vi "String to Cluster.vi"(1 "string":string) -> (0 "Correlator Initial Data 2":T1={"[0]"=1, "Channel1 Threshold Voltage (mV)"=1, "Channel1 Pulse Front"="", "Channel2 Threshold Voltage (mV)"=1, "Channel2 Pulse Front"="", "Channel3 Threshold Voltage (mV)"=1, "Channel3 Pulse Front "="", "Channel4 Threshold Voltage (mV)"=1, "Channel4 Pulse Front "="", "Single Count Enable"={"Channel1"=FALSE, "Channel2"=FALSE, "Channel3"=FALSE, "Channel4"=FALSE}, "Single Count Max"=1, "Sum Count Enable"={"Channel1"=FALSE, "Channel2"=FALSE, "Channel3"=FALSE, "Channel4"=FALSE}, "Sum Count Max"=1, "Start-Stop1 Multyplex"={"Stop Channel"="", "Start Channel"=""}, "Stop Delay 1 (ns)"=1, "Window Length 1 (ns)"=4, "Window Offset 1 (ns) "=4, "Conditional Correlation 1"="", "Histogram Bin 1"="", "Histogram Start 1 (ns) "=4, "Start-Stop2 Multyplex "={"Stop Channel"="", "Start Channel"=""}, "Stop Delay 2 (ns)"=1, "Window Length 2 (ns) "=4, "Window Offset 2 (ns) "=4, "Conditional Correlation 2"="", "Histogram Bin 2"="", "Histogram Start 2 (ns)  "=4, "Start-Stop3 Multyplex"={"Stop Channel"="", "Start Channel"=""}, "Stop Delay 3 (ns)"=1, "Window Length 3 (ns) "=4, "Window Offset 3 (ns) "=4, "Conditional Correlation 3"="", "Histogram Bin 3"="", "Histogram Start 3 (ns) "=4, "Start-Stop4 Multyplex"={"Stop Channel"="", "Start Channel"=""}, "Stop Delay 4 (ns)"=1, "Window Length 4 (ns)  "=4, "Window Offset 4 (ns) "=4, "Conditional Correlation 4"="", "Histogram Bin 4"="", "Histogram Start 4 (ns)  "=4, "Coincidence Count Enable"={"Start-Stop1"=FALSE, "Start-Stop2"=FALSE, "Start-Stop3"=FALSE, "Start-Stop4"=FALSE}, "Coincidence Count Max"=1, "Coincidence Sum Enable"={"Start-Stop1"=FALSE, "Start-Stop2"=FALSE, "Start-Stop3"=FALSE, "Start-Stop4"=FALSE}, "Coincidence Sum Max"=1, "Output Channel Enable"={"Channel1"=FALSE, "Channel2"=FALSE, "Channel3"=FALSE, "Channel4"=FALSE}, "Output Channel Inversion"={"Channel1"=FALSE, "Channel2"=FALSE, "Channel3"=FALSE, "Channel4"=FALSE, "Output"=FALSE}} {"Coincidence Sum Max" min=1 max=16777215 step=1 format="%.7e"; "Coincidence Count Max" min=1 max=16777215 step=1 format="%.7e"; "Histogram Start 4 (ns)" min=0 max=120000 step=2; "Window Offset 4 (ns)" min=0 max=120000 step=2; "Window Length 4 (ns)" min=4 max=60000 step=4; "Stop Delay 4 (ns)" min=0 max=1008 step=16; "Histogram Start 3 (ns)" min=0 max=120000 step=2; "Window Offset 3 (ns)" min=0 max=120000 step=2; "Window Length 3 (ns)" min=4 max=60000 step=4; "Stop Delay 3 (ns)" min=0 max=1008 step=16; "Histogram Start 2 (ns)" min=0 max=120000 step=2; "Window Offset 2 (ns)" min=0 max=120000 step=2; "Window Length 2 (ns)" min=4 max=60000 step=4; "Stop Delay 2 (ns)" min=0 max=1008 step=16; "Histogram Start 1 (ns)" min=0 max=120000 step=2; "Window Offset 1 (ns)" min=0 max=120000 step=2; "Window Length 1 (ns)" min=4 max=60000 step=4; "Stop Delay 1 (ns)" min=0 max=1008 step=16; "Sum Count Max" min=1 max=16777215 step=1 format="%.7e"; "Single Count Max" min=1 max=16777215 step=1 format="%.7e"; "Channel4 Threshold Voltage (mV)" min=0 max=5000 step=10; "Channel3 Threshold Voltage (mV)" min=0 max=5000 step=10; "Channel2 Threshold Voltage (mV)" min=0 max=5000 step=10; "Channel1 Threshold Voltage (mV)" min=0 max=5000 step=10; "Max Exposition Time (ms)" min=1 step=1 format="%.9e"})   [LabVIEW 2012]
panel:
  out "Output":i32[](array[numeric])
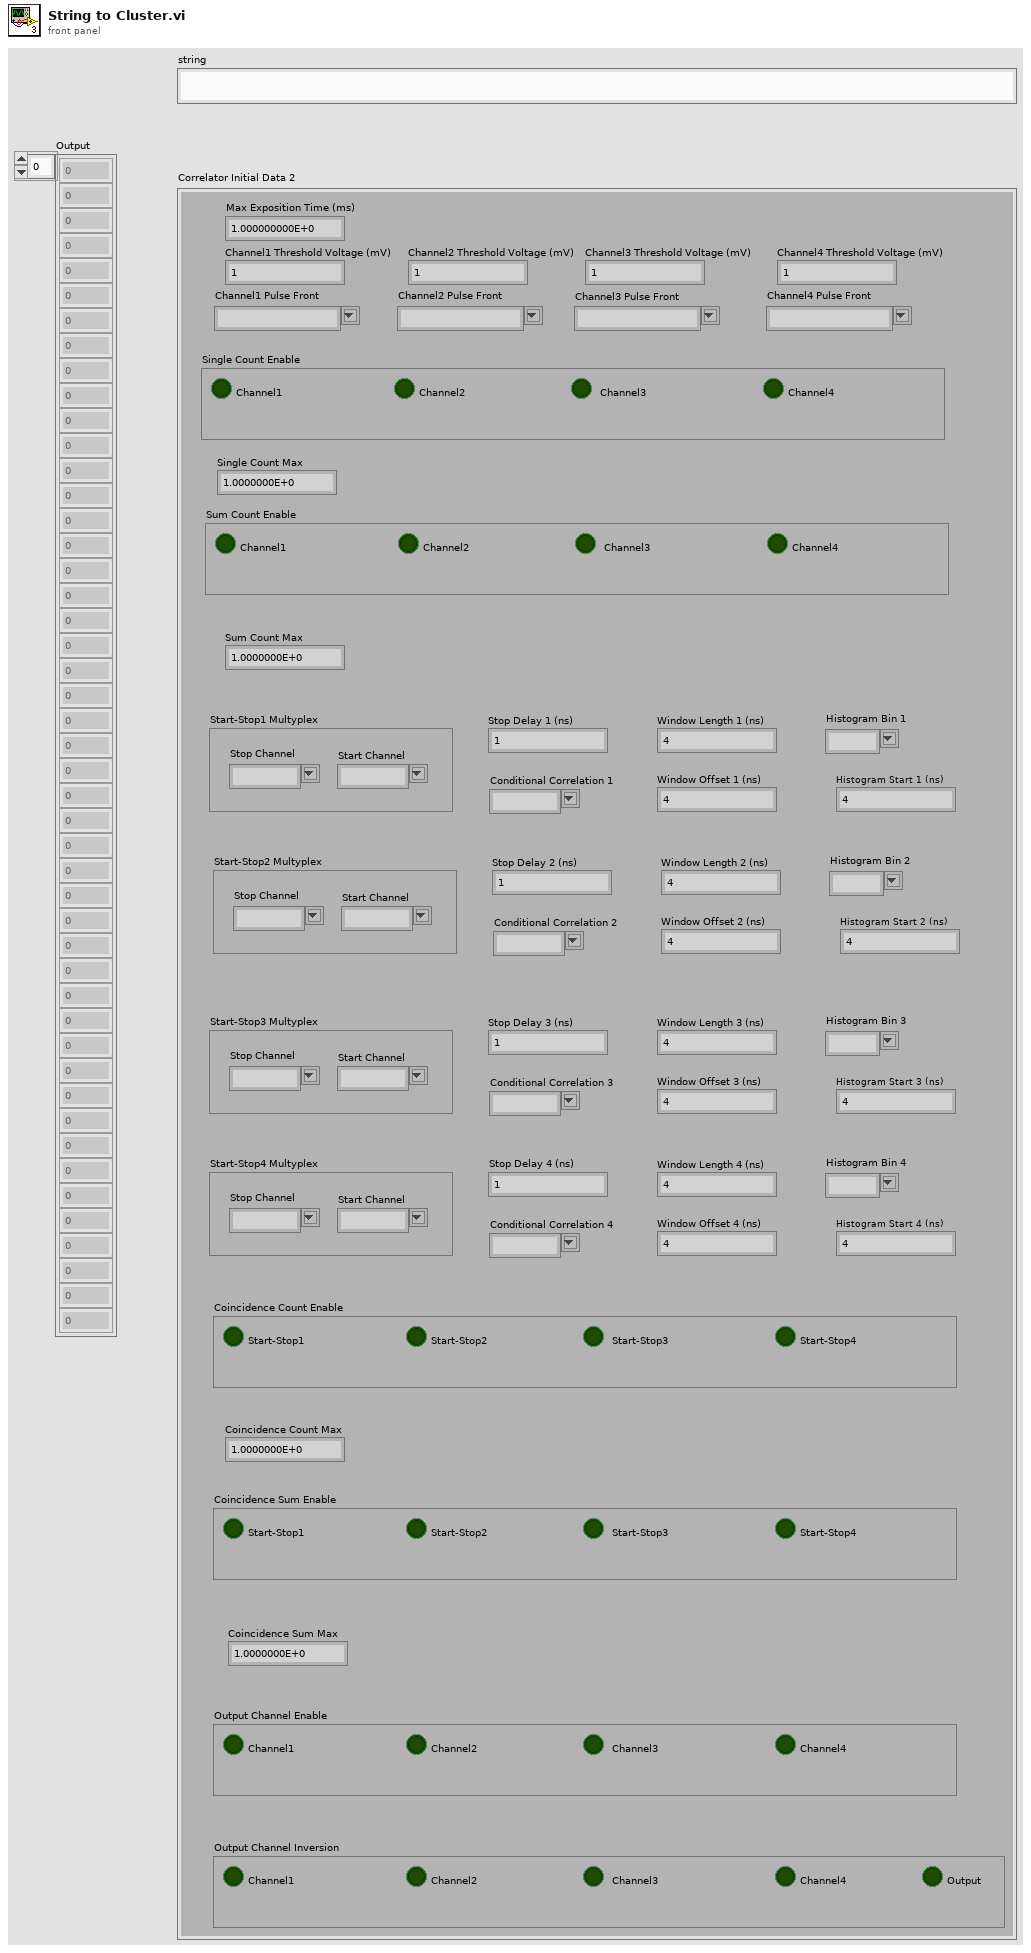
[diagram p1: front panel]
types:
  T1 = cluster{"[0]":i64, "Channel1 Threshold Voltage (mV)":i32, "Channel1 Pulse Front":string, "Channel2 Threshold Voltage (mV)":i32, "Channel2 Pulse Front":string, "Channel3 Threshold Voltage (mV)":i32, "Channel3 Pulse Front ":string, "Channel4 Threshold Voltage (mV)":i32, "Channel4 Pulse Front ":string, "Single Count Enable":cluster{"Channel1":bool, "Channel2":bool, "Channel3":bool, "Channel4":bool}, "Single Count Max":i32, "Sum Count Enable":cluster{"Channel1":bool, "Channel2":bool, "Channel3":bool, "Channel4":bool}, "Sum Count Max":i32, "Start-Stop1 Multyplex":cluster{"Stop Channel":string, "Start Channel":string}, "Stop Delay 1 (ns)":i16, "Window Length 1 (ns)":i32, "Window Offset 1 (ns) ":i32, "Conditional Correlation 1":string, "Histogram Bin 1":string, "Histogram Start 1 (ns) ":i32, "Start-Stop2 Multyplex ":cluster{"Stop Channel":string, "Start Channel":string}, "Stop Delay 2 (ns)":i16, "Window Length 2 (ns) ":i32, "Window Offset 2 (ns) ":i32, "Conditional Correlation 2":string, "Histogram Bin 2":string, "Histogram Start 2 (ns)  ":i32, "Start-Stop3 Multyplex":cluster{"Stop Channel":string, "Start Channel":string}, "Stop Delay 3 (ns)":i16, "Window Length 3 (ns) ":i32, "Window Offset 3 (ns) ":i32, "Conditional Correlation 3":string, "Histogram Bin 3":string, "Histogram Start 3 (ns) ":i32, "Start-Stop4 Multyplex":cluster{"Stop Channel":string, "Start Channel":string}, "Stop Delay 4 (ns)":i16, "Window Length 4 (ns)  ":i32, "Window Offset 4 (ns) ":i32, "Conditional Correlation 4":string, "Histogram Bin 4":string, "Histogram Start 4 (ns)  ":i32, "Coincidence Count Enable":cluster{"Start-Stop1":bool, "Start-Stop2":bool, "Start-Stop3":bool, "Start-Stop4":bool}, "Coincidence Count Max":i32, "Coincidence Sum Enable":cluster{"Start-Stop1":bool, "Start-Stop2":bool, "Start-Stop3":bool, "Start-Stop4":bool}, "Coincidence Sum Max":i32, "Output Channel Enable":cluster{"Channel1":bool, "Channel2":bool, "Channel3":bool, "Channel4":bool}, "Output Channel Inversion":cluster{"Channel1":bool, "Channel2":bool, "Channel3":bool, "Channel4":bool, "Output":bool}}
  T2 = cluster{"[0]":i64, "[1]":i64, "[2]":i64, "[3]":i64, "[4]":i64, "[5]":i64, "[6]":i64, "[7]":i64, "[8]":i64, "[9]":i64, "[10]":i64, "[11]":i64, "[12]":i64, "[13]":i64, "[14]":i64, "[15]":i64, "[16]":i64, "[17]":i64, "[18]":i64, "[19]":i64, "[20]":i64, "[21]":i64, "[22]":i64, "[23]":i64, "[24]":i64, "[25]":i64, "[26]":i64, "[27]":i64, "[28]":i64, "[29]":i64, "[30]":i64, "[31]":i64, "[32]":i64, "[33]":i64, "[34]":i64, "[35]":i64, "[36]":i64, "[37]":i64, "[38]":i64, "[39]":i64, "[40]":i64, "[41]":i64, "[42]":i64, "[43]":i64, "[44]":i64, "[45]":i64, "[46]":i64}
  T3 = cluster{"[2]":i64, "[4]":i64, "[6]":i64, "[8]":i64, "[17]":i64, "[18]":i64, "[24]":i64, "[25]":i64, "[31]":i64, "[32]":i64, "[38]":i64, "[39]":i64}
  T4 = cluster{"Boolean array[0]":bool, "Boolean array[1]":bool, "Boolean array[2]":bool, "Boolean array[3]":bool, "Boolean array[4]":bool, "Boolean array[5]":bool, "Boolean array[6]":bool, "Boolean array[7]":bool, "Boolean array[8]":bool}
  T5 = cluster{"[2]":string, "[4]":string, "[6]":string, "[8]":string, "[17]":string, "[18]":string, "[24]":string, "[25]":string, "[31]":string, "[32]":string, "[38]":string, "[39]":string}
  T6 = cluster{"Channel1":bool, "Channel2":bool, "Channel3":bool, "Channel4":bool}
  T7 = cluster{"Start Channel":string, "Stop Channel":string}
  T8 = cluster{"Boolean array[0]":bool, "Boolean array[1]":bool, "Boolean array[2]":bool, "Boolean array[3]":bool, "Boolean array[4]":bool}
  T9 = cluster{"[0]":i64, "64bit integer":i64, "[2]":string, "64bit integer":i64, "[4]":string, "64bit integer":i64, "[6]":string, "64bit integer":i64, "[8]":string, "Output Channel Enable 2":cluster{"Channel1":bool, "Channel2":bool, "Channel3":bool, "Channel4":bool}, "[10]":i64, "Output Channel Enable 2":cluster{"Channel1":bool, "Channel2":bool, "Channel3":bool, "Channel4":bool}, "[12]":i64, "Start-Stop1 Multyplex 2":cluster{"Start Channel":string, "Stop Channel":string}, "64bit integer":i64, "64bit integer":i64, "64bit integer":i64, "[17]":string, "[18]":string, "64bit integer":i64, "Start-Stop1 Multyplex 2":cluster{"Start Channel":string, "Stop Channel":string}, "64bit integer":i64, "64bit integer":i64, "64bit integer":i64, "[24]":string, "[25]":string, "64bit integer":i64, "Start-Stop1 Multyplex 2":cluster{"Start Channel":string, "Stop Channel":string}, "64bit integer":i64, "64bit integer":i64, "64bit integer":i64, "[31]":string, "[32]":string, "64bit integer":i64, "Start-Stop1 Multyplex 2":cluster{"Start Channel":string, "Stop Channel":string}, "64bit integer":i64, "64bit integer":i64, "64bit integer":i64, "[38]":string, "[39]":string, "64bit integer":i64, "Output Channel Enable 2":cluster{"Channel1":bool, "Channel2":bool, "Channel3":bool, "Channel4":bool}, "[42]":i64, "Output Channel Enable 2":cluster{"Channel1":bool, "Channel2":bool, "Channel3":bool, "Channel4":bool}, "[44]":i64, "Output Channel Enable 2":cluster{"Channel1":bool, "Channel2":bool, "Channel3":bool, "Channel4":bool}, cluster{"Boolean array[0]":bool, "Boolean array[1]":bool, "Boolean array[2]":bool, "Boolean array[3]":bool, "Boolean array[4]":bool}}
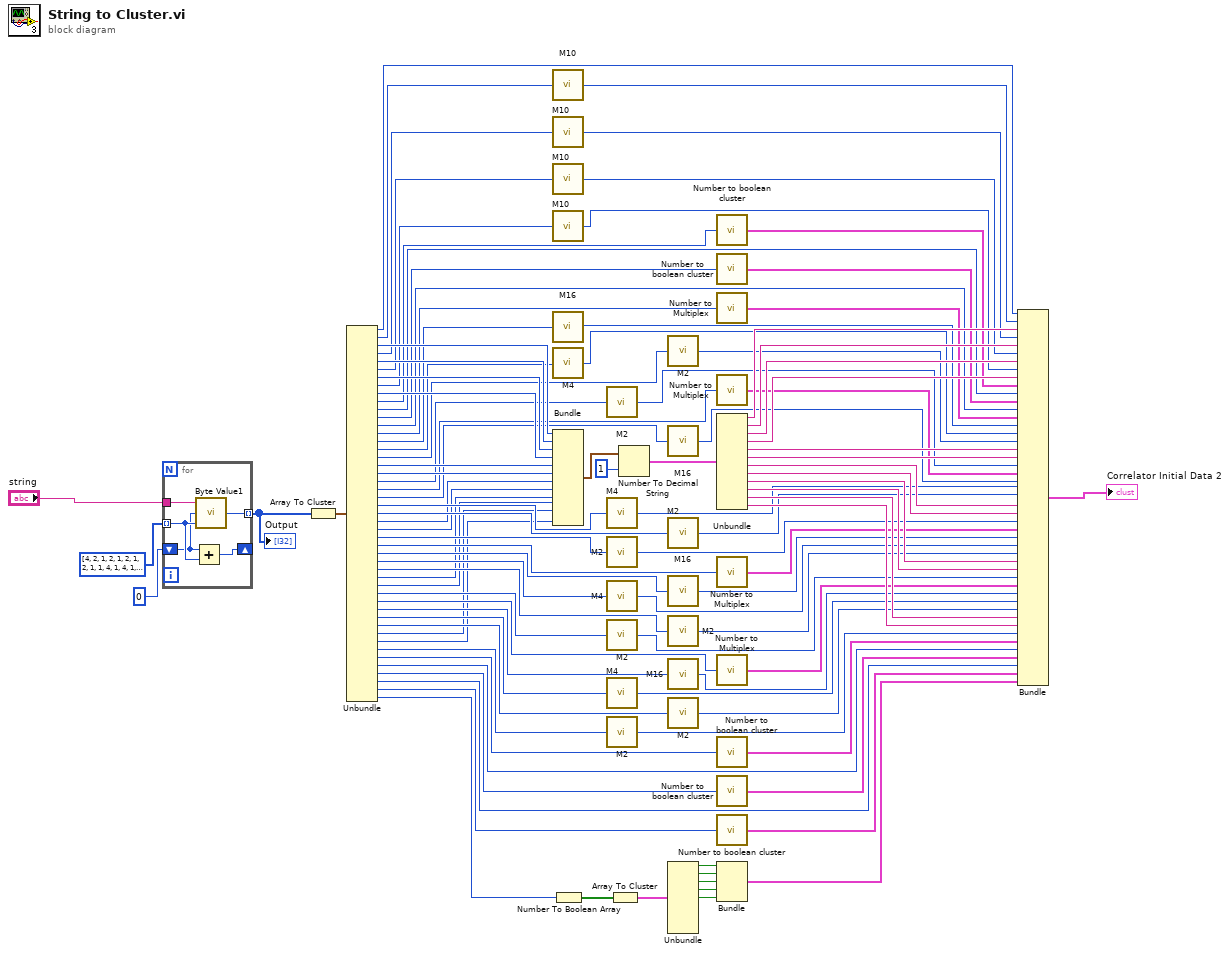
[diagram p0: block diagram]
diagram:
  n1 = for {
    tunnel: i8[] [4, 2, 1, 2, 1, 2, 1, 2, 1, 1, 4, 1, 4, 1, 1, 2, 2, 1, 1, 2, 1, 1, 2, 2, 1, 1, 2, 1, 1, 2, 2, 1, 1, 2, 1, 1, 2, 2, 1, 1, 2, 1, 4, 1, 4, 1, 1] ("Length array") -> [w109] mode=indexing
    tunnel: "string" -> [w110]
    shift-right: [w108] -> _
    shift-left: i8 0 -> [w107]
    tunnel: [w106] -> w51 mode=indexing
    n2 = Add(x=w107, y=w109) -> (x+y=w108:i8)
    n3 = call "Byte Value1.vi"("Length"=w109, "Offset"=w107, "string"=w110) -> ("Value"=w106:i64)
  }
  "Output" <- w51
  n4 = Array To Cluster(array=w51) -> (cluster=w50:T2)
  n5 = Unbundle(w50) -> ("[0]"=w49:i64, "[1]"=w48:i64, "[2]"=w47:i64, "[3]"=w46:i64, "[4]"=w45:i64, "[5]"=w44:i64, "[6]"=w43:i64, "[7]"=w42:i64, "[8]"=w41:i64, "[9]"=w40:i64, "[10]"=w39:i64, "[11]"=w38:i64, "[12]"=w37:i64, "[13]"=w36:i64, "[14]"=w35:i64, "[15]"=w34:i64, "[16]"=w33:i64, "[17]"=w32:i64, "[18]"=w31:i64, "[19]"=w30:i64, "[20]"=w29:i64, "[21]"=w28:i64, "[22]"=w27:i64, "[23]"=w26:i64, "[24]"=w25:i64, "[25]"=w24:i64, "[26]"=w23:i64, "[27]"=w22:i64, "[28]"=w21:i64, "[29]"=w20:i64, "[30]"=w19:i64, "[31]"=w18:i64, "[32]"=w17:i64, "[33]"=w16:i64, "[34]"=w15:i64, "[35]"=w13:i64, "[36]"=w12:i64, "[37]"=w11:i64, "[38]"=w10:i64, "[39]"=w9:i64, "[40]"=w8:i64, "[41]"=w7:i64, "[42]"=w6:i64, "[43]"=w5:i64, "[44]"=w4:i64, "[45]"=w3:i64, "[46]"=w2:i64)
  n6 = call "M10.vi"("x"=w48) -> ("64bit integer"=w70:i64)
  n7 = call "M10.vi"("x"=w46) -> ("64bit integer"=w69:i64)
  n8 = call "M10.vi"("x"=w44) -> ("64bit integer"=w68:i64)
  n9 = call "M10.vi"("x"=w42) -> ("64bit integer"=w67:i64)
  n10 = call "M16.vi"("x"=w35) -> ("64bit integer"=w66:i64)
  n11 = call "M4.vi"("x"=w34) -> ("64bit integer"=w65:i64)
  n12 = Bundle("[2]"=w47, "[4]"=w45, "[6]"=w43, "[8]"=w41, "[17]"=w32, "[18]"=w31, "[24]"=w25, "[25]"=w24, "[31]"=w18, "[32]"=w17, "[38]"=w10, "[39]"=w9) -> (w103:T3)  [unwired: 1 in]
  n13 = Number To Boolean Array(number=w2) -> (Boolean array=w89:bool[])
  n14 = call "M2.vi"("x"=w30) -> ("64bit integer"=w63:i64)
  n15 = call "M4.vi"("x"=w27) -> ("64bit integer"=w61:i64)
  n16 = call "M2.vi"("x"=w23) -> ("64bit integer"=w59:i64)
  n17 = call "M4.vi"("x"=w20) -> ("64bit integer"=w57:i64)
  n18 = call "M2.vi"("x"=w16) -> ("64bit integer"=w55:i64)
  n19 = call "M4.vi"("x"=w12) -> ("64bit integer"=w53:i64)
  n20 = call "M2.vi"("x"=w8) -> ("64bit integer"=w52:i64)
  n21 = Array To Cluster(array=w89) -> (cluster=w88:T4)
  n22 = Number To Decimal String(number=w103, width (-)=i16 1) -> (decimal integer string=w102:T5)
  n23 = call "M2.vi"("x"=w33) -> ("64bit integer"=w64:i64)
  n24 = call "M16.vi"("x"=w28) -> ("64bit integer"=w62:i64)
  n25 = call "M2.vi"("x"=w26) -> ("64bit integer"=w60:i64)
  n26 = call "M16.vi"("x"=w21) -> ("64bit integer"=w58:i64)
  n27 = call "M2.vi"("x"=w19) -> ("64bit integer"=w56:i64)
  n28 = call "M16.vi"("x"=w13) -> ("64bit integer"=w54:i64)
  n29 = call "M2.vi"("x"=w11) -> ("64bit integer"=w14:i64)
  n30 = Unbundle(w88) -> ("Boolean array[0]"=w87:bool, "Boolean array[1]"=w86:bool, "Boolean array[2]"=w85:bool, "Boolean array[3]"=w84:bool, "Boolean array[4]"=w83:bool)  [unwired: 4 out]
  n31 = call "Number to boolean cluster.vi"("Numeric"=w40) -> ("Output Channel Enable 2"=w78:T6)
  n32 = call "Number to boolean cluster.vi"("Numeric"=w38) -> ("Output Channel Enable 2"=w77:T6)
  n33 = call "Number to Multiplex.vi"("Numeric"=w36) -> ("Start-Stop1 Multyplex 2"=w76:T7)
  n34 = call "Number to Multiplex.vi"("Numeric"=w29) -> ("Start-Stop1 Multyplex 2"=w75:T7)
  n35 = Unbundle(w102) -> ("[2]"=w101:string, "[4]"=w100:string, "[6]"=w99:string, "[8]"=w98:string, "[17]"=w97:string, "[18]"=w96:string, "[24]"=w95:string, "[25]"=w94:string, "[31]"=w93:string, "[32]"=w92:string, "[38]"=w91:string, "[39]"=w90:string)
  n36 = call "Number to Multiplex.vi"("Numeric"=w22) -> ("Start-Stop1 Multyplex 2"=w74:T7)
  n37 = call "Number to Multiplex.vi"("Numeric"=w15) -> ("Start-Stop1 Multyplex 2"=w73:T7)
  n38 = call "Number to boolean cluster.vi"("Numeric"=w7) -> ("Output Channel Enable 2"=w79:T6)
  n39 = call "Number to boolean cluster.vi"("Numeric"=w5) -> ("Output Channel Enable 2"=w80:T6)
  n40 = call "Number to boolean cluster.vi"("Numeric"=w3) -> ("Output Channel Enable 2"=w81:T6)
  n41 = Bundle("Boolean array[0]"=w87, "Boolean array[1]"=w86, "Boolean array[2]"=w85, "Boolean array[3]"=w84, "Boolean array[4]"=w83) -> (w82:T8)  [unwired: 1 in]
  n42 = Bundle("[0]"=w49, "64bit integer"=w70, "[2]"=w101, "64bit integer"=w69, "[4]"=w100, "64bit integer"=w68, "[6]"=w99, "64bit integer"=w67, "[8]"=w98, "Output Channel Enable 2"=w78, "[10]"=w39, "Output Channel Enable 2"=w77, "[12]"=w37, "Start-Stop1 Multyplex 2"=w76, "64bit integer"=w66, "64bit integer"=w65, "64bit integer"=w64, "[17]"=w97, "[18]"=w96, "64bit integer"=w63, "Start-Stop1 Multyplex 2"=w75, "64bit integer"=w62, "64bit integer"=w61, "64bit integer"=w60, "[24]"=w95, "[25]"=w94, "64bit integer"=w59, "Start-Stop1 Multyplex 2"=w74, "64bit integer"=w58, "64bit integer"=w57, "64bit integer"=w56, "[31]"=w93, "[32]"=w92, "64bit integer"=w55, "Start-Stop1 Multyplex 2"=w73, "64bit integer"=w54, "64bit integer"=w53, "64bit integer"=w14, "[38]"=w91, "[39]"=w90, "64bit integer"=w52, "Output Channel Enable 2"=w79, "[42]"=w6, "Output Channel Enable 2"=w80, "[44]"=w4, "Output Channel Enable 2"=w81, w82) -> (→"Correlator Initial Data 2":T9)  [unwired: 1 in]
